vi "Find RPC VI For Event.vi"(10 "RPC VIs in":refnum<vi>[](array[refnum]), 11 "input event string":string=" <Server RPC Methods.RouteGuide GetFeature gRPC UE>: User Event ") -> (2 "RPC VI out":refnum<vi>, 3 "viName":string)   [LabVIEW 2019, in "gRPC Template Creation Utility.lvlib"]
uses:
  gRPC Template Creation Utility.lvlib
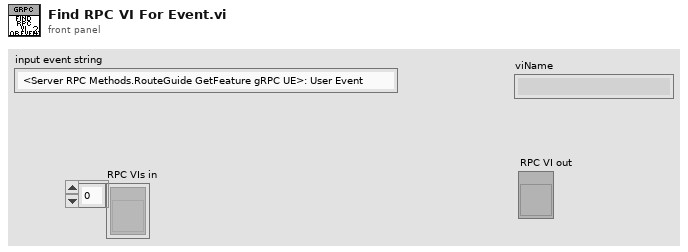
[diagram p1: front panel]
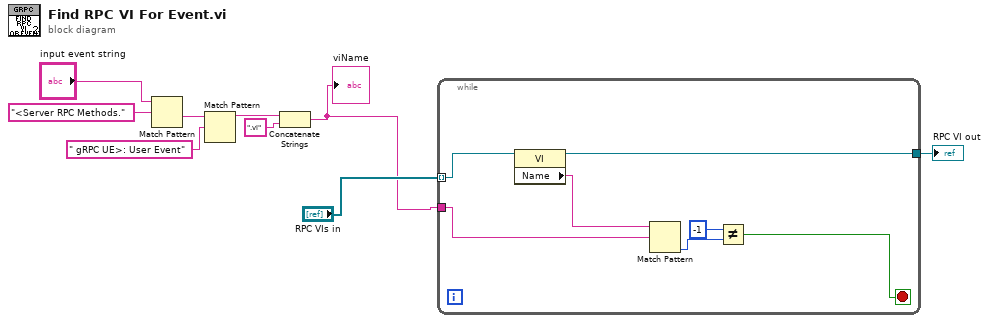
[diagram p0: block diagram]
diagram:
  n1 = Match Pattern(string="input event string", regular expression="<Server RPC Methods.") -> (after substring=w7:string)  [unwired: 1 in, 3 out]
  n2 = Match Pattern(string=w7, regular expression=" gRPC UE>: User Event") -> (before substring=w5:string)  [unwired: 1 in, 3 out]
  n3 = Concatenate Strings(w5, ".vi") -> (w2:string)
  "viName" <- w2
  n4 = while {
    tunnel: "RPC VIs in" -> [w16] mode=indexing
    tunnel: w2 -> [w12]
    tunnel: [w14] -> w1
    stop <- w15 stop-if-true
    n5 = property class="VI"(reference=w16) -> (reference out=w14:refnum<vi>, "Name"=w13:string)  [unwired: 1 in, 1 out]
    n6 = Match Pattern(string=w13, regular expression=w12) -> (offset past match=w11:i32)  [unwired: 1 in, 3 out]
    n7 = Not Equal?(x=-1, y=w11) -> (x != y?=w15:bool)
  }
  "RPC VI out" <- w1
